vi "HTTP_POST_LV20.vi"(10 "error in (no error)":errorcluster, 11 "Service Link":string) -> (1 "error out":errorcluster, 2 "Reply Body":string, 3 "Reply Header":string)   [LabVIEW 2020]
uses:
  <vilib>/httpClient/POSTBuffer.vi
  <vilib>/httpClient/LabVIEWHTTPClient.lvlib
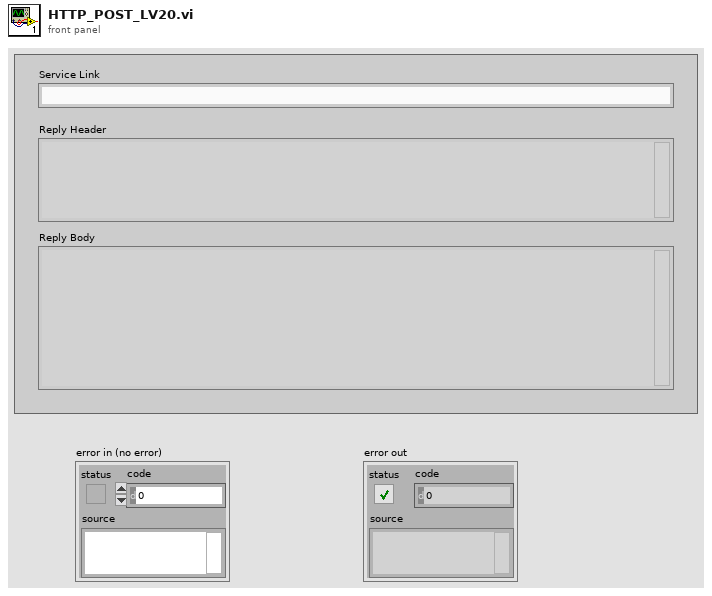
[diagram p1: front panel]
types:
  T1 = typedef "LabVIEWHTTPClient.lvlib/ClientHandle.ctl" = refnum<k1>
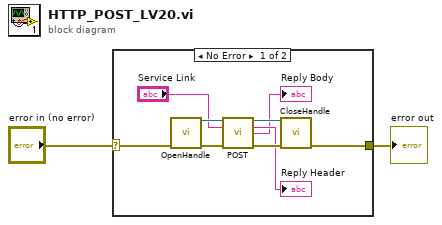
[diagram p0: block diagram]
diagram:
  n1 = case shown="No Error" "error in (no error)" {
    selector: "error in (no error)" -> [w8 w12]
    tunnel: [w5 w12] -> w1
    frame No Error {
      n2 = call <vilib>:"OpenHandle.vi"("error in (no error)"=w8) -> ("client handle out"=w11:T1, "error out"=w9:errorcluster)  [unwired: 13 in]
      n3 = call-poly <vilib>:"POST.vi"("client handle"=w11, "url"="Service Link", "error in (no error)"=w9) -> ("client handle out"=w7:T1, "headers"=→"Reply Header":string, "body"=→"Reply Body":string, "error out"=w6:errorcluster)  [unwired: 9 in]
      n4 = call <vilib>:"CloseHandle.vi"("client handle"=w7, "error in (no error)"=w6) -> ("error out"=w5:errorcluster)  [unwired: 13 in]
    }
    frame Error {
    }
  }
  "error out" <- w1
